vi "SerializableObject_To_Variant.vi"(7 "Options":T1, 8 "error IO":errorcluster, 10 "Object Name":string, 11 "Class to Serialize":refnum<class "BlueSerializable.lvclass">) -> (0 "error out":errorcluster, 3 "Vcluster":variant)   [LabVIEW 2020, in "BlueSerialization.lvlib" / "BlueSerializer.lvclass"]
uses:
  BlueSerializer.lvclass
  BlueSerializable/BlueSerializable.lvclass
  SerializeOptionsPayload.ctl
  SerializeOptions.ctl
  ClassNameCacheMap.ctl
  ClassNameObj.ctl
  GetSerializableDataAction.ctl
  GetSerializableDataCluster.ctl
  GetSerializableDataClusterClass.ctl
  SerializableDataGetDataAction.ctl
  ClassNameAndVersion.ctl
  <vilib>/Utility/EditLVLibs/LibVersion.ctl
  GetClassNameArray.vi
  SerializeSliceCalcString.vi
  BlueSerializable/SetSerializeSliceClass_StaticCommunity.vi
  GetClassNameAndVersion.vi
  GetParentClassesHiererchy.vi
  ClassNameCacheWrite.vi
  LVOOP Get Default Object Inline.vi
  GetLastCompatibleVersion.vi
  <vilib>/Utility/LVClass/Get LV Class Name.vi
  <vilib>/Utility/LVClass/Get LV Class Default Value By Name.vi
  <vilib>/Utility/EditLVLibs/LVClass/Get Mutation History.vi
  <vilib>/Utility/error.llb/Error Cluster From Error Code.vi
  <vilib>/Utility/EditLVLibs/Edit LVLibs.lvlib
  <vilib>/JDP Science/JDP Science Common Utilities/JDP Utility.lvlib
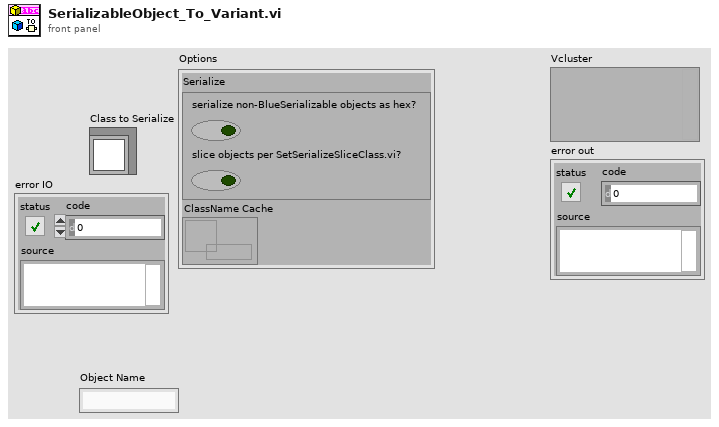
[diagram p1: front panel]
types:
  T1 = typedef "BlueSerialization.lvlib/BlueSerializer.lvclass/SerializeOptionsPayload.ctl" = cluster{"Serialize":T2, "ClassName Cache":refnum<data-value>}
  T2 = typedef "BlueSerialization.lvlib/BlueSerializer.lvclass/SerializeOptions.ctl" = cluster{"serialize non-BlueSerializable objects as hex?":bool, "slice objects per SetSerializeSliceClass.vi?":bool}
  T3 = typedef "BlueSerialization.lvlib/BlueSerializer.lvclass/GetSerializableDataAction.ctl" = enum16{"Ready For Flatten", "Unmodified Data Access"}
  T4 = typedef "BlueSerialization.lvlib/BlueSerializer.lvclass/GetSerializableDataCluster.ctl" = cluster{"Run-Mode":T3, "ClassOps":T5[], "Data":variant[], "PlaceholderData?":bool[]}
  T5 = typedef "BlueSerialization.lvlib/BlueSerializer.lvclass/GetSerializableDataClusterClass.ctl" = cluster{"Action":T6, "Class":T7}
  T6 = typedef "BlueSerialization.lvlib/BlueSerializer.lvclass/SerializableDataGetDataAction.ctl" = enum16{"Add Class", "Drop Class"}
  T7 = typedef "BlueSerialization.lvlib/BlueSerializer.lvclass/ClassNameAndVersion.ctl" = cluster{"class name":string, "Class Version":T8}
  T8 = typedef "Edit LVLibs.lvlib/LibVersion.ctl" = cluster{"Major":u16, "Minor":u16, "Fix":u16, "Build":u16}
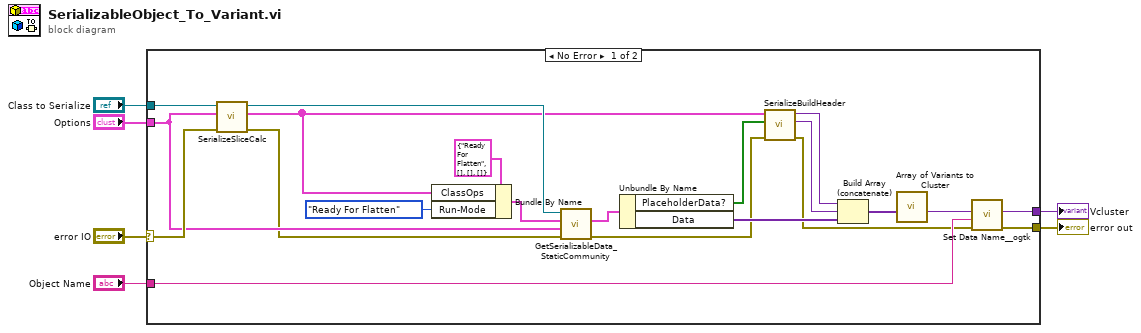
[diagram p0: block diagram]
diagram:
  n1 = case shown="No Error" "error IO" {
    selector: "error IO" -> [w25 w28]
    tunnel: "Class to Serialize" -> [w26 _]
    tunnel: [w23 w28] -> w3
    tunnel: [w24 _] -> w5
    tunnel: "Object Name" -> [w22 _]
    tunnel: "Options" -> [w15 _]
    frame No Error {
      n2 = call "SerializeSliceCalc.vi"("error in (no error)"=w25, "Options"=w15, "Class to Serialize"=w26) -> ("error out"=w14:errorcluster, "All class layers"=w12:T5[], "Class to Serialize"=w18:refnum<class "BlueSerializable.lvclass">)  [unwired: 6 in]
      n3 = Bundle By Name(cluster=T4 {"Run-Mode"=enum."Ready For Flatten", "ClassOps"=[], "Data"=[], "PlaceholderData?"=[]} ("MyData"), "ClassOps"=w12, "Run-Mode"=GetSerializableDataAction."Ready For Flatten") -> (w16:T4)
      n4 = call "GetSerializableData_StaticCommunity.vi"("error in (no error)"=w14, "Options"=w15, "Data in"=w16, "BlueSerializable in"=w18) -> ("error out"=w7:errorcluster, "Data out"=w17:T4)  [unwired: 5 in, 1 out]
      n5 = Unbundle By Name(w17) -> ("PlaceholderData?"=w11:bool[], "Data"=w19:variant[])
      n6 = call "SerializeBuildHeader.vi"("error in (no error)"=w7, "PlaceholderData?"=w11, "All class layers"=w12) -> ("error out"=w8:errorcluster, "Version header"=w10:variant, "Class header"=w9:variant)  [unwired: 6 in]
      n7 = Build Array (concatenate)(w9, w10, w19) -> (w21:variant[])
      n8 = call <vilib>:"Array of Variants to Cluster.vi"("Array of Variants"=w21) -> ("Cluster of Variants"=w20:variant)  [unwired: 10 in]
      n9 = call <userlib>:"Set Data Name__ogtk.vi"("error in (no error)"=w8, "Data Name"=w22, "Data"=w20) -> ("error out"=w23:errorcluster, "Renamed Data"=w24:variant)  [unwired: 7 in]
    }
    frame Error {
    }
  }
  "Vcluster" <- w5
  "error out" <- w3
